vi "LinearSystemId_DiffDrv_Pack_Model_Params.vi"(5 "DCMOTOR_TYPES":T3, 6 "Gear Ratio":dbl=8.0, 7 "Num Motors Per Side":i32=1, 8 "MOI-KgM2":dbl=30.0, 9 "Track Radius-m":dbl=0.8, 10 "Wheel Radius-M":dbl=0.078, 11 "Mass-Kg":dbl=200.0) -> (3 "DiffDrv_LinearSystem":T1)   [LabVIEW 2019, in "Trajectory_Library.lvlib"]
doc: "Creates a Differential Drive Train linear system from the physical parameters of the robot.. \n\nThe linear system is defined as:\n - states\n - left velocity (m/s)\n - right velocity (m/s)\n - inputs\n - left voltage (volts)\n - right voltage(volts)\n - outputs\n - left velocity (m/s)\n - right velocity (m/s)\n\nInputs:\n - DC Motor Type -- enum -- Model of the drive motor\n - Num Motors Per Side -- integer -- Number of motoes on each side of the drive\n - Mass -- double -- Robot mass (kg)\n - Wheel Radius -- double -- Radius of drive wheel (meters) Note this is radius, not diameter.\n - Track Radius -- double -- 1/2 of the distance between wheels (meters). This is effective radius which may be more than the physical radius.\n - MOI -- double -- Moment of inertia (kg m^2)\n - Gear Ratio -- double -- Drive gear ratio (Input/Output)\n\nOutput:\n - DiffDrive Linear System -- Linear System -- Created differential drive linear system"
uses:
  Trajectory_Library.lvlib
  Enum/DCMOTOR_TYPES_ENUM.ctl
  TypeDef/LINEAR_SYSTEM.ctl
  <vilib>/Analysis/Matrix/Datatypes/RealMatrix.ctl
  LinearSystem_New.vi
  MatBuilder_Create.vi
  MatBuilder_Fill.vi
  MatrixHelper_Zero.vi
  DCMotor_GetCIM.vi
  DCMotor_GetAndymark9015.vi
  DCMotor_GetAndymarkRs775_125.vi
  DCMotor_GetBag.vi
  DCMotor_GetBanebotsRs550.vi
  DCMotor_GetBanebotsRs775.vi
  DCMotor_GetFalcon500.vi
  DCMotor_GetMiniCIM.vi
  DCMotor_GetNEO.vi
  DCMotor_GetNEO550.vi
  DCMotor_GetRomiBuiltIn.vi
  DCMotor_GetVex775Pro.vi
  DCMotor_GetAndymarkAM2235A.vi
  DCMotor_GetAndymarkAM3493.vi
  DCMotor_GetFalcon500_FOC.vi
  DCMotor_GetKrakenX60.vi
  DCMotor_GetKrakenX60_FOC.vi
  DCMotor_GetNEOVortex.vi
  MatrixHelper_CoerceSize.vi
  DCMotor_New.vi
  Units_RotationsPerMinuteToRadiansPerSecond.vi
  <vilib>/Analysis/Matrix/NI_Matrix.lvlib
panel:
  # "<States,States>"
  # "<States,Inputs>"
  # "<Outputs,States>"
  # "<Outputs,Inputs>"
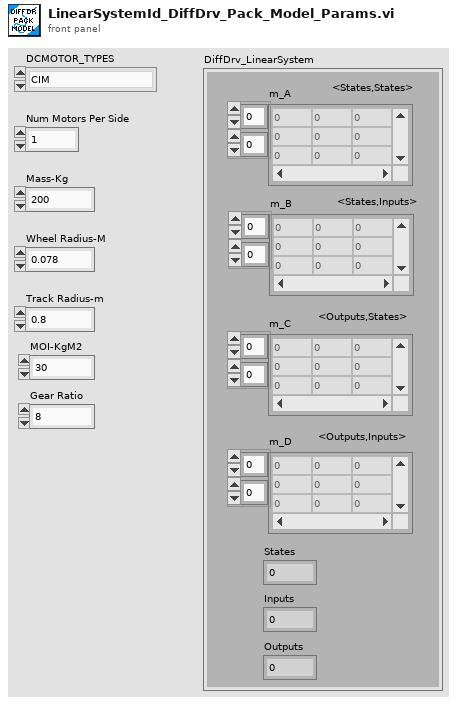
[diagram p1: front panel]
types:
  T1 = typedef "Trajectory_Library.lvlib/LINEAR_SYSTEM.ctl" = cluster{"m_A":T2, "m_B":T2, "m_C":T2, "m_D":T2, "States":i32, "Inputs":i32, "Outputs":i32}
  T2 = typedef "NI_Matrix.lvlib/RealMatrix.ctl" = dbl[][]
  T3 = typedef "Trajectory_Library.lvlib/DCMOTOR_TYPES_ENUM.ctl" = enum16{"CIM", "AndyMark 9015", "Andy Mark RS 775 125", "Bag", "BaneBots RS 550", "BaneBots RS 775", "Falcon 500", "Mini CIM", "NEO", "NEO 550", "Romi BuiltIn", "Vex 775 Pro", "Snow Blower AM 2235A", "Bosch Seat AM 3493", "Falcon 500 FOC", "Kraken X60", "Kraken X60 FOC", "NEO Vortex"}
  T4 = typedef "Trajectory_Library.lvlib/DCMOTOR.CTL" = cluster{"nominalVoltage_Volts":dbl, "StallTorque_NM":dbl, "StallCurrent_Amps":dbl, "FreeCurrent_Amps":dbl, "FreeSpeed_RadPerSec":dbl, "R_Ohms":dbl, "KvINV_RadPerSecPerVolt":dbl, "Kt_NMPerAmp":dbl, "L_H":dbl, "Jr_KgM2":dbl}
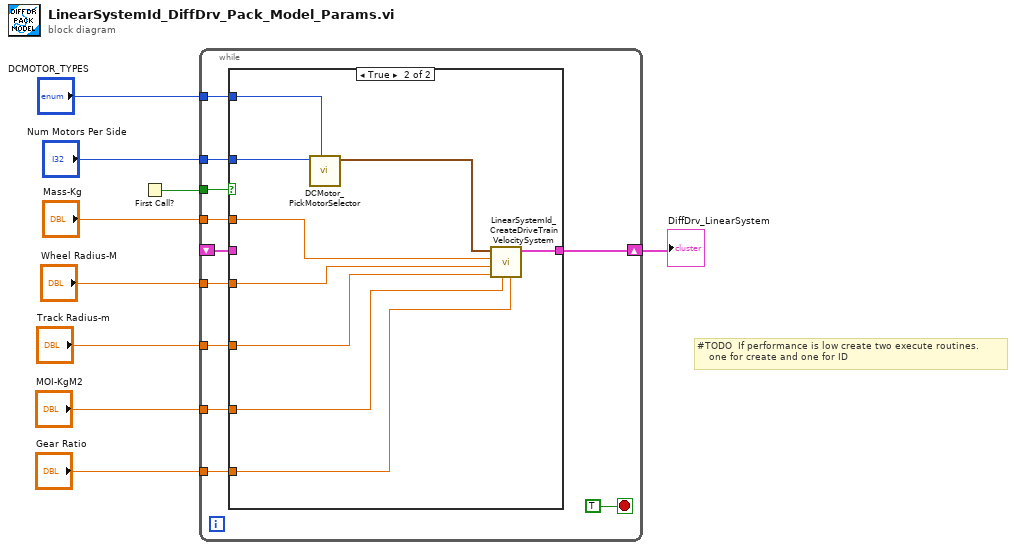
[diagram p0: block diagram]
diagram:
  # "#TODO  If performance is low create two execute routines.\n    one for create and one for ID"
  n1 = First Call?() -> (First Call?: T/F=w1:bool)
  n2 = while {
    tunnel: "DCMOTOR_TYPES" -> [w19]
    tunnel: "Num Motors Per Side" -> [w18]
    tunnel: "Mass-Kg" -> [w17]
    tunnel: "Wheel Radius-M" -> [w16]
    tunnel: "Track Radius-m" -> [w15]
    tunnel: "MOI-KgM2" -> [w14]
    tunnel: "Gear Ratio" -> [w13]
    shift-right: [w12] -> w2
    shift-left: _ -> [w10]
    tunnel: w1 -> [w11]
    stop <- TRUE stop-if-true
    n3 = case shown="True" w11 {
      tunnel: w19 -> [_ w30]
      tunnel: w18 -> [_ w29]
      tunnel: w17 -> [_ w27]
      tunnel: w16 -> [_ w26]
      tunnel: w15 -> [_ w25]
      tunnel: w14 -> [_ w24]
      tunnel: w13 -> [_ w23]
      tunnel: [w21 w22] -> w12
      tunnel: w10 -> [w21 _]
      frame False {
      }
      frame True {
        n4 = call "DCMotor_PickMotorSelector.vi"("DCMOTOR_TYPES"=w30, "Num Motors"=w29) -> ("DCMOTOR"=w28:T4)  [unwired: 9 in]
        n5 = call "LinearSystemId_CreateDriveTrainVelocitySystem.vi"("G"=w23, "JKgMetersSquared"=w24, "rbMeters"=w25, "rMeters"=w26, "MassKg"=w27, "Motor"=w28) -> ("Linearsystem"=w22:T1)  [unwired: 4 in, 1 out]
      }
    }
  }
  "DiffDrv_LinearSystem" <- w2
